vi "fo_SendFile.vi"(8 "error in (no error)":errorcluster, 10 "ServerInfo":T1={"port"=104, "AEtitle"="ME", "host"="127.0.0.1", "remoteAE"="STORESCP"}, 11 "String":string) -> (0 "error out":errorcluster)   [LabVIEW 2013, in "main.lvlib"]
uses:
  main.lvlib
  C:/Users/Simon/SkyDrive/LabView/2013/DM2020/bin/Dicom.dll
  bin/Dicom.dll
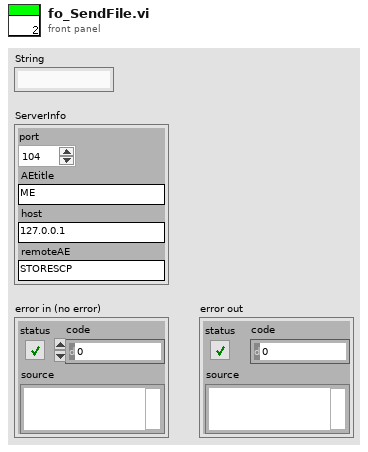
[diagram p1: front panel]
types:
  T1 = cluster{"port":i32, "AEtitle":string, "host":string, "remoteAE":string}
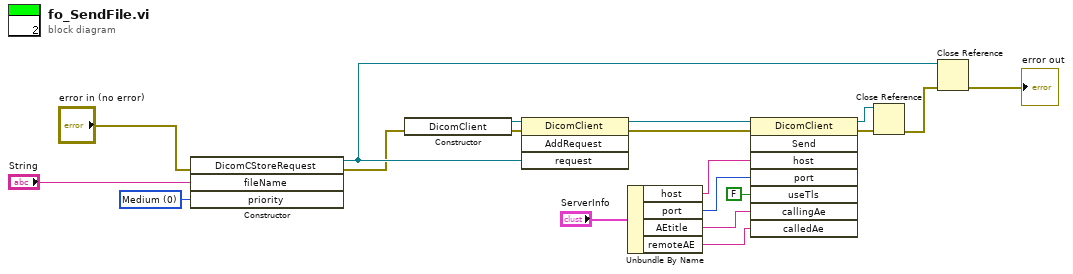
[diagram p0: block diagram]
diagram:
  w2 = u16 0 items=["Medium", "High", "Low"] ("priority")
  n1 = constructor class="DicomCStoreRequest"(error in="error in (no error)", "fileName"="String", "priority"=w2) -> (reference out=w17:refnum<k24>, error out=w4:errorcluster)  [unwired: 2 in, 3 out]
  n2 = constructor class="DicomClient"(error in=w4) -> (reference out=w3:refnum<k24>, error out=w5:errorcluster)  [unwired: 2 in, 1 out]
  n3 = invoke class="DicomClient" method="AddRequest"(reference=w3, error in=w5, "request"=w17) -> (reference out=w6:refnum<k24>, error out=w12:errorcluster)  [unwired: 1 in, 2 out]
  n4 = Unbundle By Name("ServerInfo") -> ("host"=w7:string, "port"=w8:i32, "AEtitle"=w9:string, "remoteAE"=w10:string)
  n5 = invoke class="DicomClient" method="Send"(reference=w6, error in=w12, "host"=w7, "port"=w8, "useTls"=FALSE, "callingAe"=w9, "calledAe"=w10) -> (reference out=w14:refnum<k24>, error out=w13:errorcluster)  [unwired: 1 in, 6 out]
  n6 = Close Reference(reference=w14, error in (no error)=w13) -> (error out=w15:errorcluster)
  n7 = Close Reference(reference=w17, error in (no error)=w15) -> (error out=→"error out":errorcluster)
